vi "Move Axes To Zero.vi"(7 "error in (no error)":errorcluster, 9 "Array of axes":T1[](array[typedef]), 10 "VISA in":refnum<visa-resource-name>) -> (0 "error out":errorcluster, 3 "VISA out":refnum<visa-resource-name>)   [LabVIEW 2017, in "Drivers.lvlib" / "ASI TG-1000.lvlib"]
doc: "Tells the ASI controller to move the (single) specified axis to the corresponding specified position; the equivalent of using the MOVE command. Note that it performs no checking to see if the move completes successfully."
uses:
  ASI TG-1000.lvlib
  Utility/Axis Name.ctl
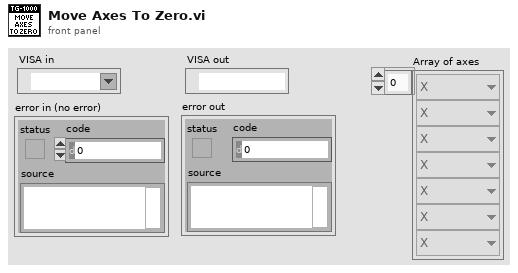
[diagram p1: front panel]
types:
  T1 = typedef "Drivers.lvlib/ASI TG-1000.lvlib/Axis Name.ctl" = enum8{"undefined", "A", "B", "C", "D", "E", "F", "G", "H", "I", "J", "K", "L", "M", "N", "O", "P", "Q", "R", "S", "T", "U", "V", "W", "X", "Y", "Z"}
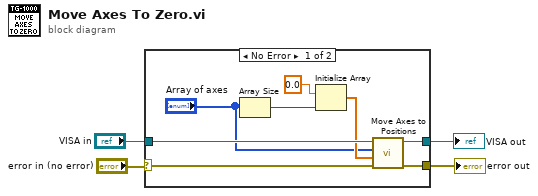
[diagram p0: block diagram]
diagram:
  n1 = case shown="No Error" "error in (no error)" {
    selector: "error in (no error)" -> [w12 w14]
    tunnel: [w11 w14] -> w3
    tunnel: "VISA in" -> [w10 w13]
    tunnel: [w9 w13] -> w1
    frame No Error {
      n2 = Array Size(array="Array of axes") -> (size(s)=w8:i32)
      n3 = Initialize Array(0.0, w8) -> (w6:dbl[])
      n4 = call "Move Axes to Positions.vi"("error in (no error)"=w12, "Array of positions [internal units]"=w6, "Array of axes"="Array of axes", "VISA in"=w10) -> ("error out"=w11:errorcluster, "VISA out"=w9:refnum<visa-resource-name>)  [unwired: 5 in]
    }
    frame Error {
    }
  }
  "VISA out" <- w1
  "error out" <- w3
